vi "Periodic Tasks.vi"(8 "error in":errorcluster) -> ()   [LabVIEW 2013]
doc: "This VI runs in parallel to other tasks. It can contain as many user-defined periodic loops as you need. These can carry out PID or other sorts of timed response."
uses:
  RefnameEnum.ctl
  <vilib>/Rock Robotics/WPI/Compressor/WPI_CompressorGetSetRefNum.vi
  Robot Global Data.vi
  <vilib>/Rock Robotics/SystemInterfaces/Utilities/FPGA_UtilitiesLED Source.ctl
  <vilib>/Rock Robotics/SystemInterfaces/Utilities/FPGA_UtilitiesLED State.ctl
  SingleSolenoidAction.ctl
  TankDriveAction.ctl
  DoubleSolenoidAction.ctl
  ShooterWrapperAction.ctl
  CollectorWrapAction.ctl
  SonarAction.ctl
  AutoAlignMode.ctl
  CatchAction.ctl
  Example_Code/PressureSensor/PressureSensorAction.ctl
  ServoAction.ctl
panel:
  out "ElevatedPassLoopTime":u32=50
  out "ElevatedPassIterations":i32=2744
  in  "CollectorMotorSpeed":dbl=1.0
  out "AutoDistanceWrapperIterations":i32=6512
  out "AutoDistanceWrapperTimer":u32=20
  in  "Slowdown":dbl=12.0 format="%#_13g"
  in  "Brake":dbl=6.0 format="%#_13g"
  in  "DesiredDistance":dbl=144.0 format="%#_13g"
  out "CatcherWrapperIterations":i32=2744
  out "CatcherWrapperTimer":u32=50
  out "CollectorWrapperTimer":u32=50
  out "CollectorWrapperIterations":i32=2743
  out "ShooterWrapperIterations":i32=2667
  out "ShooterWrapperTimer":u32=50
  out "CollectorIterations":i32=2737
  out "ClapperIterations":i32=2743
  out "RollerPneumaticIterations":i32=2743
  out "RollerMotorIterations":i32=2742
  out "FiringCylinderIterations":i32=2745
  out "KickerIterations":i32=2744
  out "SonicShifterIterations":i32=2744
  out "TankDriveIterations":i32=6485
  out "Collector Timer":u32=50
  out "Clapper Timer":u32=50
  out "Roller Pneumatic Timer":u32=50
  out "Firing Cylinder Timer":u32=50
  out "Sonic Shifter Timer":u32=50
  out "Kicker Timer":u32=50
  out "Roller Motor Timer":u32=51
  out "Tank Drive Timer":u32=21
  # "CATCH"
  # "SHOOTER WRAP"
  # "SONIC SHIFTER"
  # "TANK DRIVE"
  # "COLLECTOR WRAP"
  # "ElevatedPass"
  # "KICKER"
  # "ROLLER MOTOR"
  # "COLLECTOR ARM"
  # "FIRING CYLINDERS"
  # "AUTODISTANCE"
  # "ROLLER PNEUMATIC"
  # "CLAPPER"
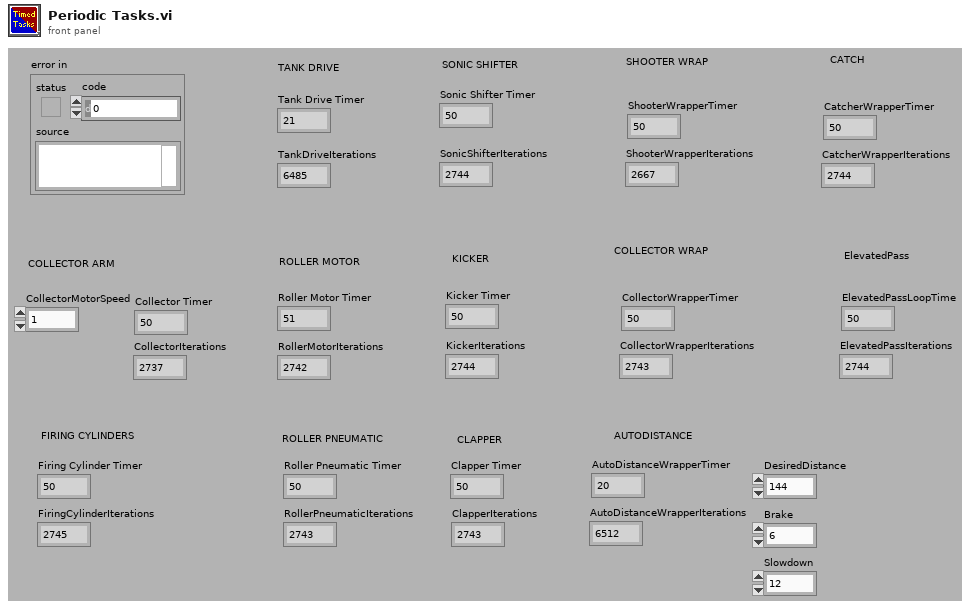
[diagram p1: front panel]
types:
  T1 = typedef "ServoAction.ctl" = enum16{"Init", "SetAngle", "GetAngle", "Disable"}
  T2 = typedef "PressureSensorAction.ctl" = enum16{"Init", "ReadValue", "Disable"}
  T3 = typedef "CatchAction.ctl" = enum16{"PreCatch", "Catch", "Stop"}
  T4 = typedef "CollectorWrapAction.ctl" = enum16{"PreCollect", "Collect", "Stop"}
  T5 = typedef "ShooterWrapperAction.ctl" = enum16{"Init", "CollectorDown", "CollectorUp"}
  T6 = typedef "ElevatedPassMode.ctl" = enum16{"Prepass", "Pass", "Stop"}
  T7 = typedef "DoubleSolenoidAction.ctl" = enum16{"Init", "Middle", "In", "Out"}
  T8 = typedef "CollectorAction.ctl" = enum16{"Init", "Raise", "Lower", "Stop", "GetStatus"}
  T9 = typedef "SingleSolenoidAction.ctl" = enum16{"Init", "SetState", "Disable"}
  T10 = typedef "TankDriveAction.ctl" = enum16{"Init", "LinearDrive", "SetValue", "Disable"}
  T11 = typedef "AutoAlignMode.ctl" = enum16{"Fullspeed", "Linear"}
  T12 = typedef "SonarAction.ctl" = enum16{"Init", "ReadValue", "Disable"}
  T13 = typedef "FPGA_UtilitiesLED State.ctl" = enum16{"Off", "On", "Toggle"}
  T14 = typedef "FPGA_UtilitiesLED Source.ctl" = enum16{"User LED", "FPGA LED"}
  T15 = typedef "RefnameEnum.ctl" = enum16{"TankDrive", "Controller1", "Controller2", "SonicShifter", "Compressor"}
  T16 = typedef "WPI_CompressorDevRef.ctl" = cluster{"DevStatus":errorcluster, "DigitalInputDevRef":T17, "RelayDevRef":T20}
  T17 = typedef "WPI_DigitalInputDevRef.ctl" = cluster{"DevStatus":errorcluster, "DIO Channel":T18, "Digital Module":T19}
  T18 = typedef "FPGA_DIOChannel.ctl" = enum8{"DIO 1", "DIO 2", "DIO 3", "DIO 4", "DIO 5", "DIO 6", "DIO 7", "DIO 8", "DIO 9", "DIO 10", "DIO 11", "DIO 12", "DIO 13", "DIO 14", "Invalid"}
  T19 = typedef "FPGA_TypedefDigitalModule.ctl" = enum16{"Digital Module 1", "Digital Module 2"}
  T20 = typedef "WPI_RelayDevRef.ctl" = cluster{"DevStatus":errorcluster, "Relay Channel":T21, "Digital Module":T19, "Relay Direction":T22}
  T21 = typedef "FPGA_DIORelayChannel.ctl" = enum8{"Relay 1", "Relay 2", "Relay 3", "Relay 4", "Relay 5", "Relay 6", "Relay 7", "Relay 8", "Invalid"}
  T22 = typedef "WPI_RelayDirection.ctl" = enum16{"Both directions", "Forward only", "Reverse only"}
  T23 = typedef "RollerAction.ctl" = enum16{"Init", "Off", "Forward", "Reverse"}
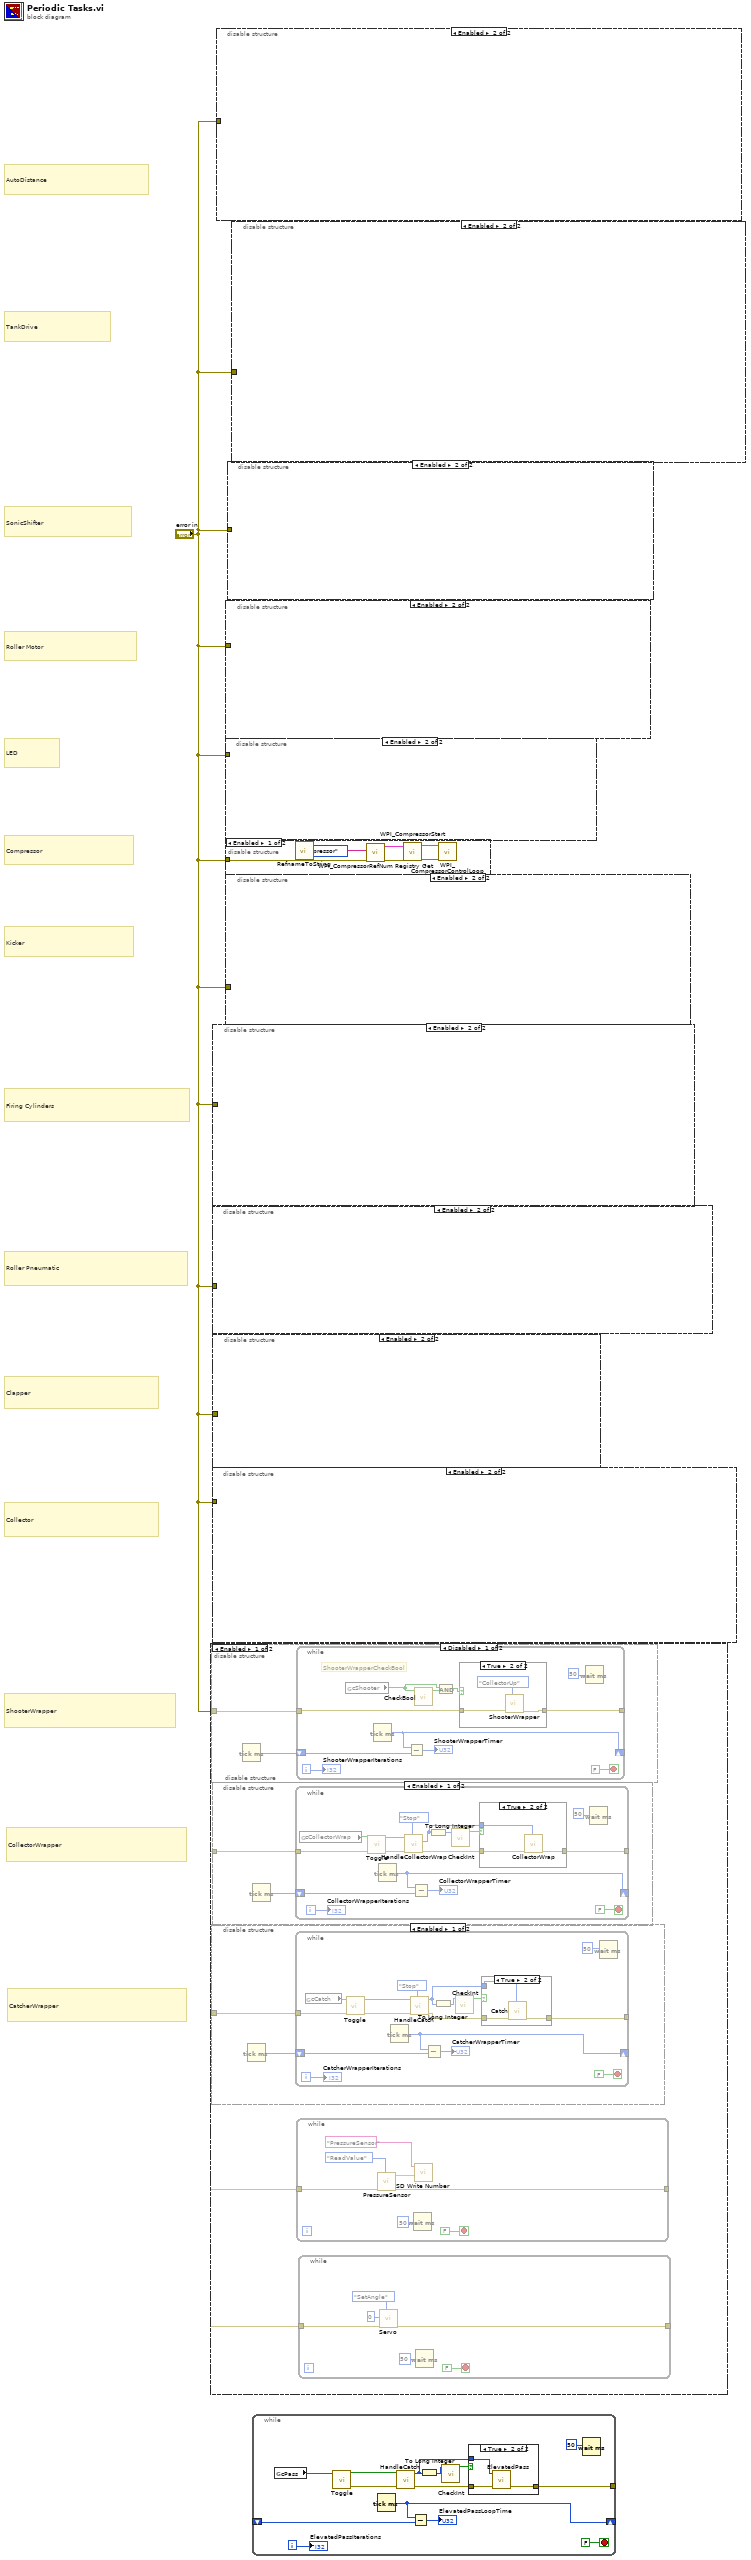
[diagram p0: block diagram]
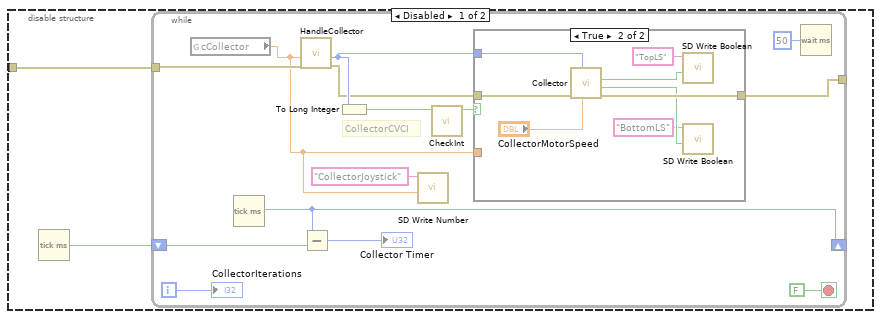
[diagram p10: hidden frame]
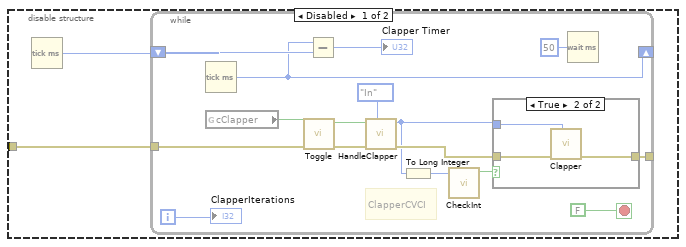
[diagram p12: hidden frame]
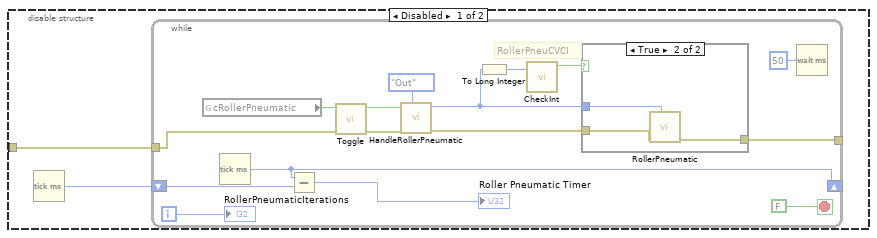
[diagram p14: hidden frame]
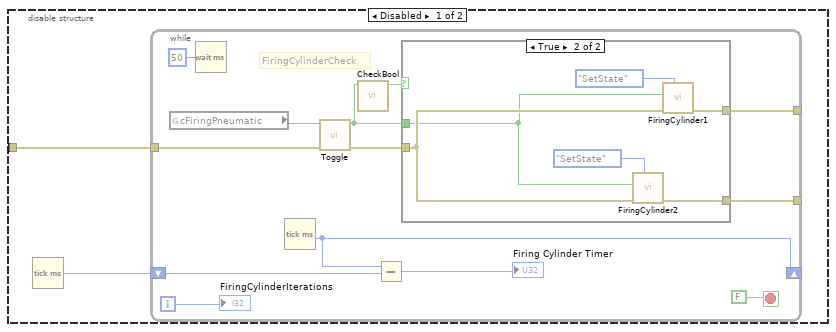
[diagram p16: hidden frame]
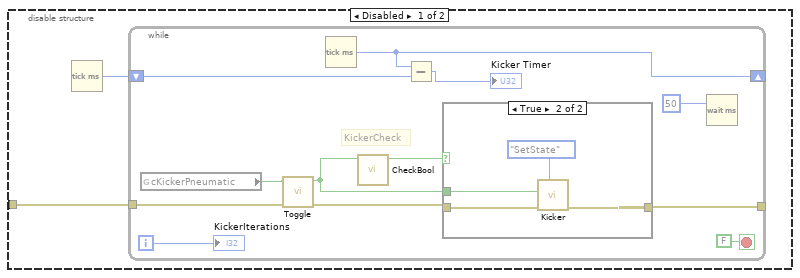
[diagram p18: hidden frame]
diagram:
  # "AutoDistance"
  # "CatcherWrapper"
  # "CollectorWrapper"
  # "ShooterWrapper"
  # "Collector"
  # "Clapper"
  # "Roller Pneumatic"
  # "Firing Cylinders"
  # "Kicker"
  # "Compressor"
  # "Roller Motor"
  # "SonicShifter"
  # "LED"
  # "TankDrive"
  n1 = disable-structure shown="Disabled" {
    disable-tunnel: "error in" -> [w2 _]
    frame Disabled {
      n2 = disable-structure shown="Enabled" {
        disable-tunnel: w2 -> [w61 _]
        frame Enabled {
          n3 = Tick Count (ms)() -> (millisecond timer value=w60:u32)
          n4 = while {
            tunnel: w61 -> [w68]
            shift-right: [w69] -> _
            shift-left: w60 -> [w70]
            tunnel: [w67] -> _
            i -> [w65]
            stop <- FALSE stop-if-true
            # "ShooterWrapperCheckBool"
            n5 = global read "Robot Global Data.vi" "cShooter"() -> (w62:bool)
            n6 = Tick Count (ms)() -> (millisecond timer value=w69:u32)
            n7 = Subtract(x=w69, y=w70) -> (x-y=→"ShooterWrapperTimer":u32)
            n8 = call "CheckBool.vi"("Input Boolean"=w62) -> ("Boolean Changed?"=w64:bool)  [unwired: 10 in]
            n9 = And(x=w62, y=w64) -> (x .and. y?=w63:bool)
            n10 = case shown="True" w63 {
              tunnel: w68 -> [w73 w76]
              tunnel: [w73 w75] -> w67
              frame False {
              }
              frame True {
                n11 = call "ShooterWrapper.vi"("Action"=ShooterWrapperAction."CollectorUp", "error in"=w76) -> ("error out"=w75:errorcluster)  [unwired: 8 in]
              }
            }
            n12 = Wait (ms)(milliseconds to wait=u32 50) -> ()  [unwired: 1 out]
            "ShooterWrapperIterations" <- w65
          }
        }
        frame Disabled {
        }
      }
      n13 = disable-structure shown="Enabled" {
        disable-tunnel: w2 -> [w17 _]
        frame Enabled {
          n14 = Tick Count (ms)() -> (millisecond timer value=w16:u32)
          n15 = while {
            tunnel: w17 -> [w33]
            tunnel: [w30] -> _
            shift-right: [w25] -> _
            shift-left: w16 -> [w26]
            i -> [w27]
            stop <- FALSE stop-if-true
            n16 = global read "Robot Global Data.vi" "cCatch"() -> (w32:bool)
            n17 = call "Toggle.vi"("error in"=w33, "RawInput"=w32) -> ("error out"=w23:errorcluster, "ToggleState"=w19:bool)  [unwired: 8 in]
            n18 = Tick Count (ms)() -> (millisecond timer value=w25:u32)
            n19 = call "HandleCatch.vi"(7:CatchAction."Stop" ("InitState"), "error in (no error)"=w23, "Toggle?"=w19) -> ("error out"=w22:errorcluster, "ElevatedPassMode"=w20:T6)  [unwired: 7 in]
            n20 = Subtract(x=w25, y=w26) -> (x-y=→"CatcherWrapperTimer":u32)
            n21 = To Long Integer(number=w20) -> (32bit integer=w21:i32)
            n22 = call "CheckInt.vi"("Integer"=w21) -> ("Changed?"=w31:bool)  [unwired: 10 in]
            n23 = case shown="True" w31 {
              tunnel: w22 -> [w34 w37]
              tunnel: [w34 w36] -> w30
              tunnel: w20 -> [_ w35]
              frame False {
              }
              frame True {
                n24 = call "Catch.vi"("Action"=w35, "error in (no error)"=w37) -> ("error out"=w36:errorcluster)  [unwired: 9 in]
              }
            }
            n25 = Wait (ms)(milliseconds to wait=u32 50) -> ()  [unwired: 1 out]
            "CatcherWrapperIterations" <- w27
          }
        }
        frame Disabled {
        }
      }
      n26 = disable-structure shown="Enabled" {
        disable-tunnel: w2 -> [w39 _]
        frame Enabled {
          n27 = Tick Count (ms)() -> (millisecond timer value=w38:u32)
          n28 = while {
            tunnel: w39 -> [w48]
            shift-right: [w52] -> _
            shift-left: w38 -> [w53]
            tunnel: [w51] -> _
            i -> [w49]
            stop <- FALSE stop-if-true
            n29 = global read "Robot Global Data.vi" "cCollectorWrap"() -> (w47:bool)
            n30 = call "Toggle.vi"("error in"=w48, "RawInput"=w47) -> ("error out"=w46:errorcluster, "ToggleState"=w44:bool)  [unwired: 8 in]
            n31 = Tick Count (ms)() -> (millisecond timer value=w52:u32)
            n32 = call "HandleCollectorWrap.vi"("InitState"=CollectorWrapAction."Stop", "error in (no error)"=w46, "Toggle?"=w44) -> ("error out"=w43:errorcluster, "State"=w40:T4)  [unwired: 7 in]
            n33 = Subtract(x=w52, y=w53) -> (x-y=→"CollectorWrapperTimer":u32)
            n34 = To Long Integer(number=w40) -> (32bit integer=w41:i32)
            n35 = call "CheckInt.vi"("Integer"=w41) -> ("Changed?"=w42:bool)  [unwired: 10 in]
            n36 = case shown="True" w42 {
              tunnel: [w56 w59] -> w51
              tunnel: w43 -> [w56 w58]
              tunnel: w40 -> [_ w57]
              frame False {
              }
              frame True {
                n37 = call "CollectorWrap.vi"("Action"=w57, "error in"=w58) -> ("error out"=w59:errorcluster)  [unwired: 9 in]
              }
            }
            n38 = Wait (ms)(milliseconds to wait=u32 50) -> ()  [unwired: 1 out]
            "CollectorWrapperIterations" <- w49
          }
        }
        frame Disabled {
        }
      }
      n39 = while {
        tunnel: w2 -> [w14]
        tunnel: [w13] -> _
        stop <- FALSE stop-if-true
        n40 = call "PressureSensor.vi"("Action"=PressureSensorAction."ReadValue", "error in (no error)"=w14) -> ("error out"=w13:errorcluster, "Pressure"=w9:dbl)  [unwired: 8 in]
        n41 = Wait (ms)(milliseconds to wait=u32 50) -> ()  [unwired: 1 out]
        n42 = call <vilib>:"SD Write Number.vi"("Numeric"=w9, "Name"="PressureSensor") -> ()  [unwired: 8 in, 2 out]
      }
      n43 = while {
        tunnel: [w7] -> _
        tunnel: w2 -> [w5]
        stop <- FALSE stop-if-true
        n44 = call "Servo.vi"("Action"=ServoAction."SetAngle", "error in (no error)"=w5, "Angle (deg)"=0) -> ("error out"=w7:errorcluster)  [unwired: 7 in, 1 out]
        n45 = Wait (ms)(milliseconds to wait=u32 50) -> ()  [unwired: 1 out]
      }
    }
    frame Enabled {
    }
  }
  n46 = disable-structure shown="Enabled" {
    disable-tunnel: "error in" -> [w78 _]
    frame Disabled {
      n47 = Tick Count (ms)() -> (millisecond timer value=w77:u32)
      n48 = while {
        tunnel: w78 -> [w82]
        shift-right: [w91] -> _
        shift-left: w77 -> [w90]
        tunnel: [w84] -> _
        i -> [w83]
        stop <- FALSE stop-if-true
        # "RollerPneuCVCI"
        n49 = global read "Robot Global Data.vi" "cRollerPneumatic"() -> (w80:bool)
        n50 = Tick Count (ms)() -> (millisecond timer value=w91:u32)
        n51 = Subtract(x=w91, y=w90) -> (x-y=→"Roller Pneumatic Timer":u32)
        n52 = call "Toggle.vi"("error in"=w82, "RawInput"=w80) -> ("error out"=w81:errorcluster, "ToggleState"=w79:bool)  [unwired: 8 in]
        n53 = call "HandleRollerPneumatic.vi"("InitState"=DoubleSolenoidAction."Out", "error in (no error)"=w81, "Toggle?"=w79) -> ("error out"=w85:errorcluster, "State"=w86:T7)  [unwired: 7 in]
        n54 = To Long Integer(number=w86) -> (32bit integer=w88:i32)
        n55 = call "CheckInt.vi"("Integer"=w88) -> ("Changed?"=w87:bool)  [unwired: 10 in]
        n56 = case shown="True" w87 {
          tunnel: w86 -> [_ w98]
          tunnel: w85 -> [w95 w97]
          tunnel: [w95 w96] -> w84
          frame False {
          }
          frame True {
            n57 = call "RollerPneumatic.vi"("State"=w98, "Error in"=w97) -> ("Error out"=w96:errorcluster)  [unwired: 9 in]
          }
        }
        n58 = Wait (ms)(milliseconds to wait=u32 50) -> ()  [unwired: 1 out]
        "RollerPneumaticIterations" <- w83
      }
    }
    frame Enabled {
    }
  }
  n59 = disable-structure shown="Enabled" {
    disable-tunnel: "error in" -> [w100 _]
    frame Disabled {
      n60 = Tick Count (ms)() -> (millisecond timer value=w99:u32)
      n61 = while {
        tunnel: w100 -> [w113]
        shift-right: [w110] -> _
        shift-left: w99 -> [w111]
        tunnel: [w104] -> _
        i -> [w103]
        stop <- FALSE stop-if-true
        # "CollectorCVCI"
        n62 = global read "Robot Global Data.vi" "cCollector"() -> (w101:dbl)
        n63 = Tick Count (ms)() -> (millisecond timer value=w110:u32)
        n64 = call "HandleCollector.vi"("error in"=w113, "JoystickValue"=w101) -> ("error out"=w105:errorcluster, "CollectorEnum Input"=w106:T8)  [unwired: 8 in]
        n65 = Subtract(x=w110, y=w111) -> (x-y=→"Collector Timer":u32)
        n66 = To Long Integer(number=w106) -> (32bit integer=w108:i32)
        n67 = call <vilib>:"SD Write Number.vi"("Numeric"=w101, "Name"="CollectorJoystick") -> ()  [unwired: 8 in, 2 out]
        n68 = call "CheckInt.vi"("Integer"=w108) -> ("Changed?"=w107:bool)  [unwired: 10 in]
        n69 = case shown="True" w107 {
          tunnel: w106 -> [_ w123]
          tunnel: w105 -> [w115 w122]
          tunnel: [w115 w121] -> w104
          tunnel: w101 -> [_ _]
          frame False {
          }
          frame True {
            n70 = call "Collector.vi"("MotorSpeed"="CollectorMotorSpeed", "Action"=w123, "Error in"=w122) -> ("Error out"=w121:errorcluster, "Lower Triggered?"=w119:bool, "Upper Triggered?"=w120:bool)  [unwired: 6 in]
            n71 = call <vilib>:"SD Write Boolean.vi"("Boolean"=w120, "Name"="TopLS") -> ()  [unwired: 8 in, 2 out]
            n72 = call <vilib>:"SD Write Boolean.vi"("Boolean"=w119, "Name"="BottomLS") -> ()  [unwired: 8 in, 2 out]
          }
        }
        n73 = Wait (ms)(milliseconds to wait=u32 50) -> ()  [unwired: 1 out]
        "CollectorIterations" <- w103
      }
    }
    frame Enabled {
    }
  }
  n74 = disable-structure shown="Enabled" {
    disable-tunnel: "error in" -> [w125 _]
    frame Disabled {
      n75 = Tick Count (ms)() -> (millisecond timer value=w124:u32)
      n76 = while {
        tunnel: w125 -> [w130]
        shift-right: [w136] -> _
        shift-left: w124 -> [w135]
        tunnel: [w133] -> _
        tunnel: [w132] -> _
        i -> [w126]
        stop <- FALSE stop-if-true
        # "FiringCylinderCheck"
        n77 = global read "Robot Global Data.vi" "cFiringPneumatic"() -> (w131:bool)
        n78 = Wait (ms)(milliseconds to wait=u32 50) -> ()  [unwired: 1 out]
        n79 = Tick Count (ms)() -> (millisecond timer value=w136:u32)
        n80 = call "Toggle.vi"("error in"=w130, "RawInput"=w131) -> ("error out"=w129:errorcluster, "ToggleState"=w127:bool)  [unwired: 8 in]
        n81 = call "CheckBool.vi"("Input Boolean"=w127) -> ("Boolean Changed?"=w128:bool)  [unwired: 10 in]
        n82 = Subtract(x=w136, y=w135) -> (x-y=→"Firing Cylinder Timer":u32)
        n83 = case shown="True" w128 {
          tunnel: w129 -> [w139 w141]
          tunnel: [w139 w143] -> w133
          tunnel: [w139 w142] -> w132
          tunnel: w127 -> [_ w140]
          frame False {
          }
          frame True {
            n84 = call "FiringCylinder2.vi"("Action"=SingleSolenoidAction."SetState", "error in (no error)"=w141, "Actuate?"=w140) -> ("error out"=w142:errorcluster)  [unwired: 8 in]
            n85 = call "FiringCylinder1.vi"("Action"=SingleSolenoidAction."SetState", "error in (no error)"=w141, "Actuate?"=w140) -> ("error out"=w143:errorcluster)  [unwired: 8 in]
          }
        }
        "FiringCylinderIterations" <- w126
      }
    }
    frame Enabled {
    }
  }
  n86 = disable-structure shown="Enabled" {
    disable-tunnel: "error in" -> [w147 _]
    frame Disabled {
      n87 = Tick Count (ms)() -> (millisecond timer value=w146:u32)
      n88 = while {
        tunnel: w147 -> [w152]
        shift-right: [w148] -> _
        shift-left: w146 -> [w149]
        tunnel: [w158] -> _
        i -> [w154]
        stop <- FALSE stop-if-true
        # "ClapperCVCI"
        n89 = Tick Count (ms)() -> (millisecond timer value=w148:u32)
        n90 = global read "Robot Global Data.vi" "cClapper"() -> (w153:bool)
        n91 = call "Toggle.vi"("error in"=w152, "RawInput"=w153) -> ("error out"=w151:errorcluster, "ToggleState"=w150:bool)  [unwired: 8 in]
        n92 = Subtract(x=w148, y=w149) -> (x-y=→"Clapper Timer":u32)
        n93 = call "HandleClapper.vi"("InitState"=DoubleSolenoidAction."In", "error in (no error)"=w151, "Toggle?"=w150) -> ("error out"=w159:errorcluster, "State"=w156:T7)  [unwired: 7 in]
        n94 = To Long Integer(number=w156) -> (32bit integer=w157:i32)
        n95 = call "CheckInt.vi"("Integer"=w157) -> ("Changed?"=w155:bool)  [unwired: 10 in]
        n96 = case shown="True" w155 {
          tunnel: w156 -> [_ w167]
          tunnel: w159 -> [w164 w166]
          tunnel: [w164 w165] -> w158
          frame False {
          }
          frame True {
            n97 = call "Clapper.vi"("State"=w167, "Error in"=w166) -> ("Error out"=w165:errorcluster)  [unwired: 9 in]
          }
        }
        n98 = Wait (ms)(milliseconds to wait=u32 50) -> ()  [unwired: 1 out]
        "ClapperIterations" <- w154
      }
    }
    frame Enabled {
    }
  }
  n99 = disable-structure shown="Enabled" {
    disable-tunnel: "error in" -> [w169 _]
    frame Disabled {
      n100 = Tick Count (ms)() -> (millisecond timer value=w168:u32)
      n101 = while {
        tunnel: w169 -> [w179]
        tunnel: [w178] -> _
        shift-right: [w173] -> _
        shift-left: w168 -> [w174]
        i -> [w175]
        stop <- FALSE stop-if-true
        n102 = global read "Robot Global Data.vi" "cAutoDistance"() -> (w171:bool)
        n103 = call "CheckBool.vi"("Input Boolean"=w171) -> ("Boolean Changed?"=w170:bool)  [unwired: 10 in]
        n104 = case shown="True" w171 {
          tunnel: w179 -> [w182 w198]
          tunnel: [w181 w195] -> w178
          tunnel: w170 -> [w180 _]
          frame False {
            n105 = case shown="True" w180 {
              tunnel: w182 -> [w183 w187]
              tunnel: [w183 w186] -> w181
              frame False {
              }
              frame True {
                w185 = 0.0 ("LeftDesired")
                n106 = call "TankDrive.vi"("DriveAction"=TankDriveAction."SetValue", "error in (no error)"=w187, "RightDesired"=w185, "LeftDesired"=w185) -> ("error out"=w186:errorcluster)  [unwired: 6 in, 1 out]
              }
            }
          }
          frame True {
            n107 = call "Sonar.vi"("Action"=SonarAction."ReadValue", "error in (no error)"=w198) -> ("error out"=w192:errorcluster, "distance"=w194:dbl)  [unwired: 8 in]
            n108 = call <vilib>:"SD Write Number.vi"("Numeric"=w194, "Name"="FrontSonar") -> ()  [unwired: 8 in, 2 out]
            n109 = call "AutoDistance.vi"("Mode"=AutoAlignMode."Linear", "Slowdown"="Slowdown", "Brake"="Brake", "DesiredDistance"="DesiredDistance", "CurrentDistance"=w194) -> ("TankDriveRight"=w188:dbl, "TankDriveLeft"=w189:dbl, "Finished"=w191:bool)  [unwired: 4 in]
            n110 = call "TankDrive.vi"("DriveAction"=TankDriveAction."SetValue", "error in (no error)"=w192, "RightDesired"=w188, "LeftDesired"=w189) -> ("error out"=w195:errorcluster)  [unwired: 6 in, 1 out]
            n111 = call <vilib>:"SD Write Boolean.vi"("Boolean"=w191, "Name"="AutoDistanceDone?") -> ()  [unwired: 8 in, 2 out]
          }
        }
        n112 = Tick Count (ms)() -> (millisecond timer value=w173:u32)
        n113 = Subtract(x=w173, y=w174) -> (x-y=→"AutoDistanceWrapperTimer":u32)
        n114 = Wait (ms)(milliseconds to wait=u32 20) -> ()  [unwired: 1 out]
        "AutoDistanceWrapperIterations" <- w175
      }
    }
    frame Enabled {
    }
  }
  n115 = disable-structure shown="Enabled" {
    disable-tunnel: "error in" -> [w203 _]
    frame Disabled {
      n116 = while {
        tunnel: w203 -> [w205]
        tunnel: [w204] -> _
        stop <- FALSE stop-if-true
        # "This global is written to in the Autonomous and Teleop VIs"
        n117 = call <vilib>:"WPI_UtilitiesFRC LEDs.vi"("error in (no error)"=w205, "State"=FPGA_UtilitiesLED_State."Toggle", "LED Type"=FPGA_UtilitiesLED_Source."User LED") -> ("error out"=w204:errorcluster)  [unwired: 8 out]
        n118 = global read "Robot Global Data.vi" "LED toggle rate (ms)"() -> (w206:u32)
        n119 = Wait (ms)(milliseconds to wait=w206) -> ()  [unwired: 1 out]
      }
    }
    frame Enabled {
    }
  }
  n120 = disable-structure shown="Enabled" {
    disable-tunnel: "error in" -> [w216 _]
    frame Enabled {
      n121 = call "RefnameToString.vi"("Enum"=RefnameEnum."Compressor") -> ("Refname"=w213:string)
      n122 = call <vilib>:"WPI_CompressorRefNum Registry Get.vi"("error in (no error)"=w216, "refnum name"=w213) -> ("error out"=w215:errorcluster, "CompressorDevRef"=w211:T16)  [unwired: 8 in]
      n123 = call <vilib>:"WPI_CompressorStart.vi"("error in (no error)"=w215, "CompressorDevRef"=w211) -> ("error out"=w214:errorcluster, "CompressorDevRef"=w210:T16)  [unwired: 8 in]
      n124 = call <vilib>:"WPI_CompressorControlLoop.vi"("error in (no error)"=w214, "CompressorDevRef"=w210) -> ()  [unwired: 10 in]
    }
    frame Disabled {
    }
  }
  n125 = disable-structure shown="Enabled" {
    disable-tunnel: "error in" -> [w218 _]
    frame Disabled {
      n126 = Tick Count (ms)() -> (millisecond timer value=w217:u32)
      n127 = while {
        tunnel: w218 -> [w229]
        shift-right: [w227] -> _
        shift-left: w217 -> [w225]
        tunnel: [w221] -> _
        i -> [w219]
        stop <- FALSE stop-if-true
        # "RollerMotorCVCI"
        n128 = Tick Count (ms)() -> (millisecond timer value=w227:u32)
        n129 = global read "Robot Global Data.vi" "cRoller"() -> (w228:dbl)
        n130 = call "RollerProcessInput.vi"("error in"=w229, "JoystickValue"=w228) -> ("error out"=w222:errorcluster, "StateOut"=w220:T23)  [unwired: 8 in]
        n131 = Subtract(x=w227, y=w225) -> (x-y=→"Roller Motor Timer":u32)
        n132 = To Long Integer(number=w220) -> (32bit integer=w224:i32)
        n133 = call "CheckInt.vi"("Integer"=w224) -> ("Changed?"=w223:bool)  [unwired: 10 in]
        n134 = case shown="True" w223 {
          tunnel: w220 -> [_ w235]
          tunnel: w222 -> [w232 w234]
          tunnel: [w232 w233] -> w221
          frame False {
          }
          frame True {
            n135 = call "Roller Motor Control.vi"("Action"=w235, "Error in"=w234) -> ("Error out"=w233:errorcluster)  [unwired: 9 in]
          }
        }
        n136 = Wait (ms)(milliseconds to wait=u32 50) -> ()  [unwired: 1 out]
        "RollerMotorIterations" <- w219
      }
    }
    frame Enabled {
    }
  }
  n137 = disable-structure shown="Enabled" {
    disable-tunnel: "error in" -> [w237 _]
    frame Disabled {
      n138 = Tick Count (ms)() -> (millisecond timer value=w236:u32)
      n139 = while {
        tunnel: w237 -> [w243]
        shift-right: [w245] -> _
        shift-left: w236 -> [w247]
        tunnel: [w244] -> _
        i -> [w238]
        stop <- FALSE stop-if-true
        # "KickerCheck"
        n140 = global read "Robot Global Data.vi" "cKickerPneumatic"() -> (w241:bool)
        n141 = call "Toggle.vi"("error in"=w243, "RawInput"=w241) -> ("error out"=w242:errorcluster, "ToggleState"=w239:bool)  [unwired: 8 in]
        n142 = Tick Count (ms)() -> (millisecond timer value=w245:u32)
        n143 = call "CheckBool.vi"("Input Boolean"=w239) -> ("Boolean Changed?"=w240:bool)  [unwired: 10 in]
        n144 = Subtract(x=w245, y=w247) -> (x-y=→"Kicker Timer":u32)
        n145 = case shown="True" w240 {
          tunnel: w242 -> [w250 w252]
          tunnel: [w250 w253] -> w244
          tunnel: w239 -> [_ w251]
          frame False {
          }
          frame True {
            n146 = call "Kicker.vi"("Action"=SingleSolenoidAction."SetState", "error in (no error)"=w252, "Actuate?"=w251) -> ("error out"=w253:errorcluster)  [unwired: 8 in]
          }
        }
        n147 = Wait (ms)(milliseconds to wait=u32 50) -> ()  [unwired: 1 out]
        "KickerIterations" <- w238
      }
    }
    frame Enabled {
    }
  }
  n148 = disable-structure shown="Enabled" {
    disable-tunnel: "error in" -> [w256 _]
    frame Disabled {
      n149 = Tick Count (ms)() -> (millisecond timer value=w255:u32)
      n150 = while {
        tunnel: w256 -> [w261]
        shift-right: [w265] -> _
        shift-left: w255 -> [w266]
        tunnel: [w263] -> _
        i -> [w258]
        stop <- FALSE stop-if-true
        n151 = global read "Robot Global Data.vi" "cSonicShifter"() -> (w262:bool)
        n152 = call "Toggle.vi"("error in"=w261, "RawInput"=w262) -> ("error out"=w260:errorcluster, "ToggleState"=w257:bool)  [unwired: 8 in]
        n153 = Tick Count (ms)() -> (millisecond timer value=w265:u32)
        n154 = Subtract(x=w265, y=w266) -> (x-y=→"Sonic Shifter Timer":u32)
        n155 = call "CheckBool.vi"("Input Boolean"=w257) -> ("Boolean Changed?"=w259:bool)  [unwired: 10 in]
        n156 = case shown="True" w259 {
          tunnel: [w269 w272] -> w263
          tunnel: w260 -> [w269 w271]
          tunnel: w257 -> [_ w270]
          frame False {
          }
          frame True {
            n157 = call "SonicShifter.vi"("Action"=SingleSolenoidAction."SetState" ("Mode"), "error in (no error)"=w271, "Actuate?"=w270) -> ("error out"=w272:errorcluster)  [unwired: 8 in]
          }
        }
        n158 = Wait (ms)(milliseconds to wait=u32 50) -> ()  [unwired: 1 out]
        "SonicShifterIterations" <- w258
      }
    }
    frame Enabled {
    }
  }
  n159 = disable-structure shown="Enabled" {
    disable-tunnel: "error in" -> [w275 _]
    frame Disabled {
      n160 = Tick Count (ms)() -> (millisecond timer value=w274:u32)
      n161 = while {
        tunnel: w275 -> [w280]
        shift-right: [w299] -> _
        shift-left: w274 -> [w298]
        tunnel: [w291] -> _
        i -> [w288]
        stop <- FALSE stop-if-true
        n162 = global read "Robot Global Data.vi" "cReverseDrive"() -> (w287:bool)
        n163 = global read "Robot Global Data.vi" "cStraightDrive"() -> (w284:bool)
        n164 = global read "Robot Global Data.vi" "cTankDriveRight"() -> (w296:dbl)
        n165 = global read "Robot Global Data.vi" "cTankDriveLeft"() -> (w295:dbl)
        n166 = global read "Robot Global Data.vi" "cHalfDrive"() -> (w283:bool)
        n167 = Tick Count (ms)() -> (millisecond timer value=w299:u32)
        n168 = Wait (ms)(milliseconds to wait=u32 20) -> ()  [unwired: 1 out]
        n169 = call "Toggle.vi"("RawInput"=w287) -> ("ToggleState"=w281:bool)  [unwired: 9 in, 1 out]
        n170 = Subtract(x=w299, y=w298) -> (x-y=→"Tank Drive Timer":u32)
        n171 = call "Sonar.vi"("Action"=SonarAction."ReadValue", "error in (no error)"=w280) -> ("error out"=w278:errorcluster, "distance"=w276:dbl)  [unwired: 8 in]
        n172 = call "HandleDrive.vi"("Deadzone"=0.15, "RightMotor"=w296, "LeftMotor"=w295) -> ("Enqueue?"=w294:bool, "RightMotor"=w292:dbl, "LeftMotor"=w293:dbl)  [unwired: 6 in]
        n173 = call <vilib>:"SD Write Boolean.vi"("Boolean"=w281, "Name"="ReverseDrive") -> ()  [unwired: 8 in, 2 out]
        n174 = call <vilib>:"SD Write Number.vi"("error in"=w278, "Numeric"=w276, "Name"="FrontSonar") -> ()  [unwired: 7 in, 2 out]
        n175 = call <vilib>:"SD Write Boolean.vi"("Boolean"=w284, "Name"="StraightDrive") -> ()  [unwired: 8 in, 2 out]
        n176 = call <vilib>:"SD Write Boolean.vi"("Boolean"=w283, "Name"="HalfDrive") -> ()  [unwired: 8 in, 2 out]
        n177 = case shown="True" w294 {
          tunnel: w293 -> [_ w310]
          tunnel: w292 -> [_ w309]
          tunnel: [w301 w308] -> w291
          tunnel: w280 -> [w301 w307]
          tunnel: w281 -> [_ w304]
          tunnel: w283 -> [_ w303]
          tunnel: w284 -> [_ w302]
          frame False {
          }
          frame True {
            w317 = 0.0  # Cutoff
            n178 = call "HalfDrive.vi"("RightDrive in"=w309, "LeftDrive in"=w310, "HalfDrive"=w303) -> ("RightDrive out"=w316:dbl, "LeftDrive out"=w315:dbl)  [unwired: 7 in]
            n179 = call "StraightDrive.vi"("RightDrive in"=w316, "LeftDrive in"=w315, "StraightDrive"=w302) -> ("RightDrive out"=w313:dbl, "LeftDrive out"=w314:dbl)  [unwired: 7 in]
            n180 = call "ReverseDrive.vi"("cReverseDrive"=w304, "Right"=w313, "Left"=w314) -> ("Right"=w311:dbl, "Left"=w312:dbl)  [unwired: 7 in]
            n181 = call <vilib>:"SD Read Number.vi"("Name"="MaxMotorChange") -> ("Numeric"=w305:dbl)  [unwired: 8 in, 2 out]
            n182 = call "TankDrive.vi"("MaxMotorChangeForward"=w305, "Cutoff"=w317, "DriveAction"=TankDriveAction."SetValue", "error in (no error)"=w307, "RightDesired"=w311, "LeftDesired"=w312) -> ("error out"=w308:errorcluster)  [unwired: 4 in, 1 out]
          }
        }
        "TankDriveIterations" <- w288
      }
    }
    frame Enabled {
    }
  }
  n183 = while {
    tunnel: [w331] -> _
    shift-right: [w326] -> _
    shift-left: _ -> [w327]
    i -> [w328]
    stop <- FALSE stop-if-true
    n184 = global read "Robot Global Data.vi" "cPass"() -> (w319:bool)
    n185 = call "Toggle.vi"("RawInput"=w319) -> ("error out"=w324:errorcluster, "ToggleState"=w321:bool)  [unwired: 9 in]
    n186 = Tick Count (ms)() -> (millisecond timer value=w326:u32)
    n187 = call "HandleCatch.vi"("error in (no error)"=w324, "Toggle?"=w321) -> ("error out"=w323:errorcluster, "ElevatedPassMode"=w320:T6)  [unwired: 8 in]
    n188 = Subtract(x=w326, y=w327) -> (x-y=→"ElevatedPassLoopTime":u32)
    n189 = To Long Integer(number=w320) -> (32bit integer=w322:i32)
    n190 = call "CheckInt.vi"("Integer"=w322) -> ("Changed?"=w332:bool)  [unwired: 10 in]
    n191 = case shown="True" w332 {
      tunnel: w323 -> [w333 w336]
      tunnel: [w333 w335] -> w331
      tunnel: w320 -> [_ w334]
      frame False {
      }
      frame True {
        n192 = call "ElevatedPass.vi"("error in (no error)"=w336, "ElevatedPassMode"=w334) -> ("error out"=w335:errorcluster)  [unwired: 9 in]
      }
    }
    n193 = Wait (ms)(milliseconds to wait=u32 50) -> ()  [unwired: 1 out]
    "ElevatedPassIterations" <- w328
  }
